vi "E18_NodosDePropiedad.vi"() -> ()   [LabVIEW 2026]
panel:
  out "Elapsed Time (s)":dbl
  out "Running":bool
  out "Waveform Chart":cluster{dbl, dbl, dbl}(graph)
  in  "stop":bool
  out "Alarma 02":string
  out "Alarma 01":string
  in  "Parámetros":cluster{"Ganancia K":dbl, "Uo":dbl}
  in  "Medición Simulada":dbl(slide) scale=0.0..20.0
  out "Nivel de tanque":dbl(slide) scale=0.0..10.0
  # "Nivel en m^3"
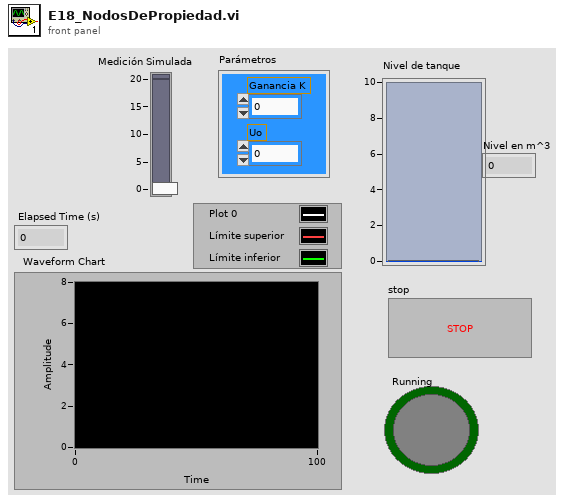
[diagram p1: front panel]
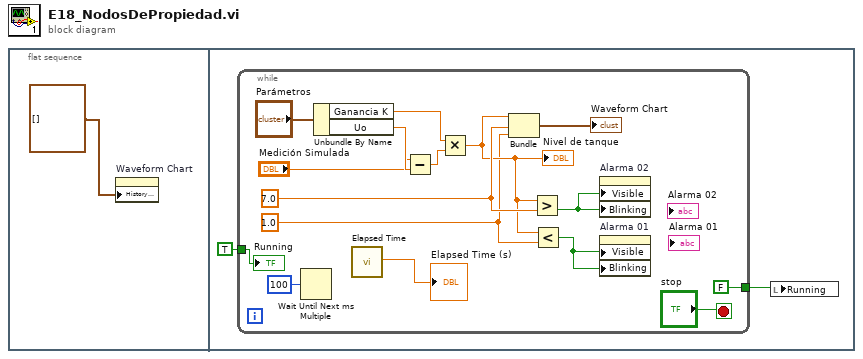
[diagram p0: block diagram]
diagram:
  n1 = flat-sequence {
    frame #0 {
      n2 = property on="Waveform Chart" class="WFChart (strict)"("History Data"=cluster{dbl, dbl, dbl}[] []) -> ()  [unwired: 2 in, 2 out]
    }
    frame #1 {
      n3 = while {
        tunnel: TRUE -> [w8]
        tunnel: [FALSE] -> w2
        stop <- "stop" stop-if-true
        w9 = 1.0
        w11 = 7.0
        n4 = Wait Until Next ms Multiple(millisecond multiple=u32 100) -> ()  [unwired: 1 out]
        n5 = Unbundle By Name("Parámetros") -> ("Ganancia K"=w14:dbl, "Uo"=w17:dbl)
        n6 = call "Elapsed Time"() -> ("Elapsed Time (s)"=→"Elapsed Time (s)":dbl)  [unwired: 12 in, 7 out]
        n7 = Subtract(x="Medición Simulada", y=w17) -> (x-y=w15:dbl)
        n8 = Multiply(x=w14, y=w15) -> (x*y=w10:dbl)
        "Nivel de tanque" <- w10
        n9 = Bundle(w10, w11, w9) -> (→"Waveform Chart":cluster{dbl, dbl, dbl})  [unwired: 1 in]
        n10 = Greater?(x=w10, y=w11) -> (0:w4:bool)
        n11 = Less?(x=w10, y=w9) -> (x < y?=w5:bool)
        n12 = property on="Alarma 02" class="Str"("Visible"=w4, "Blinking"=w4) -> ()  [unwired: 2 in, 2 out]
        n13 = property on="Alarma 01" class="Str"("Visible"=w5, "Blinking"=w5) -> ()  [unwired: 2 in, 2 out]
        "Running" <- w8
      }
      n14 = local write "Running"(w2) -> ()
    }
  }
